vi "huffman_encoder.vi"(9 "Python version":string, 10 "module path":path=path "D:/Thesis Pak Pri/huffman_encoder.py", 11 "bit_array":i16[](array[numeric])) -> (3 "return value":i32[](array[numeric]))   [LabVIEW 2018]
panel:
  out "error out":errorcluster
  in  "error in (no error)":errorcluster
  in  "function name":string="encode_huffman_image"
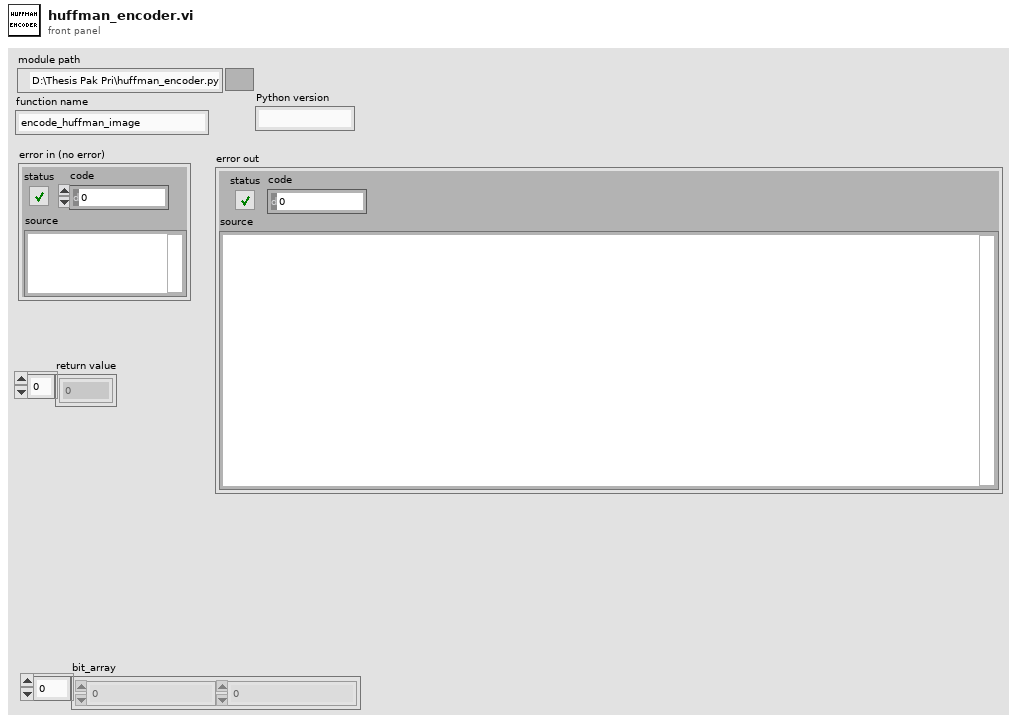
[diagram p1: front panel]
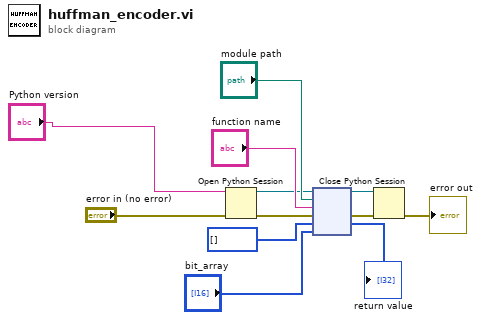
[diagram p0: block diagram]
diagram:
  n1 = Open Python Session(python version="Python version", 3:"error in (no error)") -> (session out=w10:refnum<k35>, error out=w9:errorcluster)  [unwired: 1 in]
  n2 = node(w10, "module path", "function name", w9, i32[] [], "bit_array") -> (w8:refnum<k35>, w7:errorcluster, →"return value":i32[])  [unwired: 1 in, 2 out]
  n3 = Close Python Session(session in=w8, error in=w7) -> (11:→"error out":errorcluster)
